vi "公式未完成.vi"() -> ()   [LabVIEW 2018]
panel:
  out "第二个解":cdb
  out "第一个解":cdb
  in  "D":dbl
  in  "C":dbl
  in  "B":dbl
  in  "A":dbl
  # "AX2+BX+C=D"
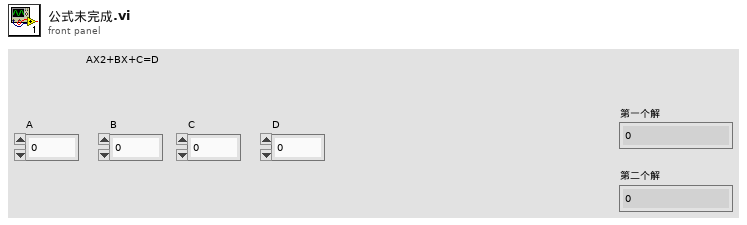
[diagram p1: front panel]
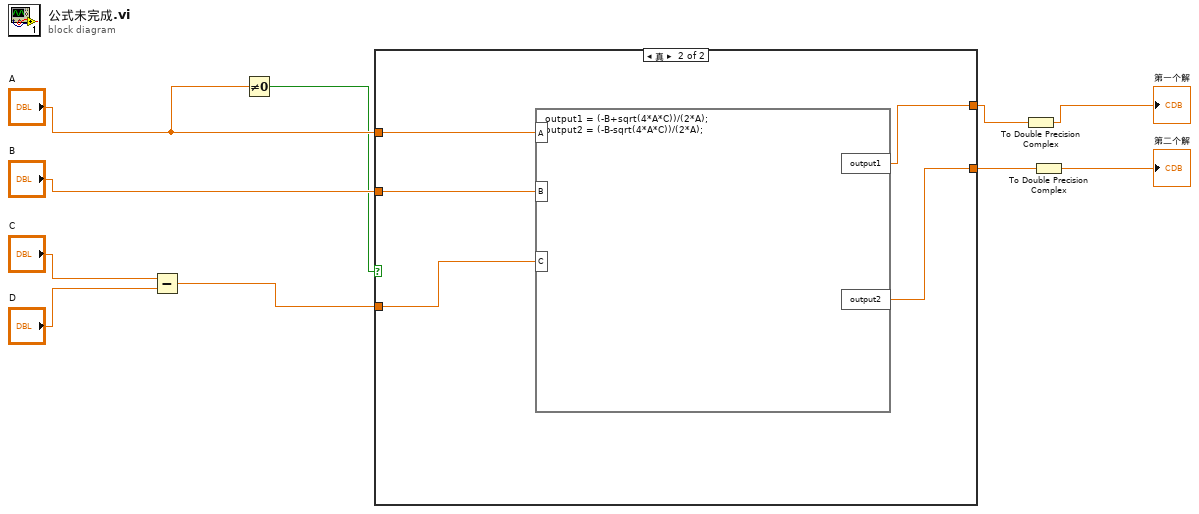
[diagram p0: block diagram]
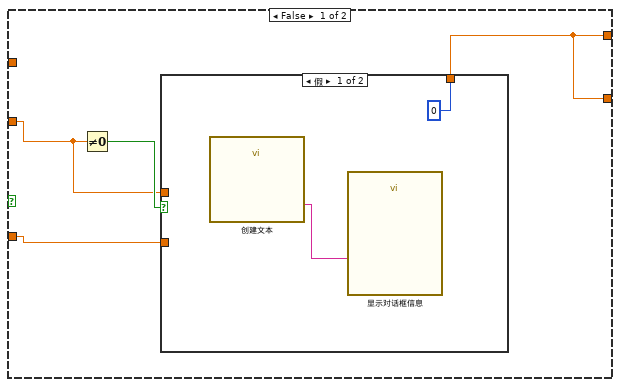
[diagram p2: hidden frame]
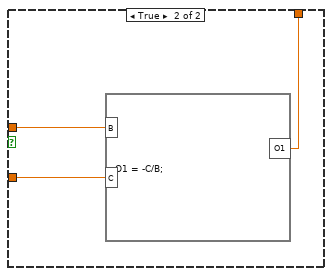
[diagram p3: hidden frame]
diagram:
  n1 = Subtract(x="C", y="D") -> (x-y=w8:dbl)
  n2 = Not Equal To 0?(x="A") -> (x != 0?=w5:bool)
  n3 = case shown="真" w5 {
    tunnel: w8 -> [w12 w24]
    tunnel: "A" -> [_ w23]
    tunnel: "B" -> [w13 w22]
    tunnel: [w11 w21] -> w4
    tunnel: [w11 w20] -> w2
    frame False {
      n4 = Not Equal To 0?(x=w13) -> (x != 0?=w14:bool)
      n5 = case shown="假" w14 {
        tunnel: w13 -> [_ w19]
        tunnel: w12 -> [_ w18]
        tunnel: [0 w17] -> w11
        frame False {
          n6 = call "创建文本"() -> ("Result"=w16:string)  [unwired: 14 in, 1 out]
          n7 = call "显示对话框信息"("Message"=w16) -> ()  [unwired: 9 in, 2 out]
        }
        frame True {
          n8 = formula code="O1 = -C/B;"("B"=w19, "C"=w18) -> ("O1"=w17:dbl)
        }
      }
    }
    frame True {
      n9 = formula code="output1 = (-B+sqrt(4*A*C))/(2*A);\noutput2 = (-B-sqrt(4*A*C))/(2*A);"("A"=w23, "B"=w22, "C"=w24) -> ("output1"=w21:dbl, "output2"=w20:dbl)
    }
  }
  n10 = To Double Precision Complex(1:w4) -> (0:→"第一个解":cdb)
  n11 = To Double Precision Complex(1:w2) -> (0:→"第二个解":cdb)
